vi "Config Axis.vi"(0 "X-Axis configuration":T1, 5 "Y-Axis configuration":T1, 7 "Z-Axis configuration":T1, 11 "error in (no error)":errorcluster) -> (15 "error out":errorcluster)   [LabVIEW 2024, in "GRBL 1.1.lvlib"]
doc: "X-axis travel resolution: X-axis travel resolution in steps per millimeter. (step/mm)\nY-axis travel resolution: Y-axis travel resolution in steps per millimeter. (step/mm)\nZ-axis travel resolution: Z-axis travel resolution in steps per millimeter. (step/mm)\nX-axis maximum rate: X-axis maximum rate. Used as G0 rapid rate. (mm/min)\nY-axis maximum rate: Y-axis maximum rate. Used as G0 rapid rate. (mm/min)\nZ-axis maximum rate: Z-axis maximum rate. Used as G0 rapid rate. (mm/min)\nX-axis acceleration: X-axis acceleration. Used for motion planning to not exceed motor torque and lose steps. (mm/sec^2)\nY-axis acceleration: Y-axis acceleration. Used for motion planning to not exceed motor torque and lose steps. (mm/sec^2)\nZ-axis acceleration: Z-axis acceleration. Used for motion planning to not exceed motor torque and lose steps. (mm/sec^2)\nX-axis maximum travel: Maximum X-axis travel distance from homing switch. Determines valid machine space for soft-limits and homing search distances. (millimeters)\nY-axis maximum travel: Maximum Y-axis travel distance from homing switch. Determines valid machine space for soft-limits and homing search distances. (millimeters)\nZ-axis maximum travel: Maximum Z-axis travel distance from homing switch. Determines valid machine space for soft-limits and homing search distances. (millimeters)"
uses:
  GRBL 1.1.lvlib
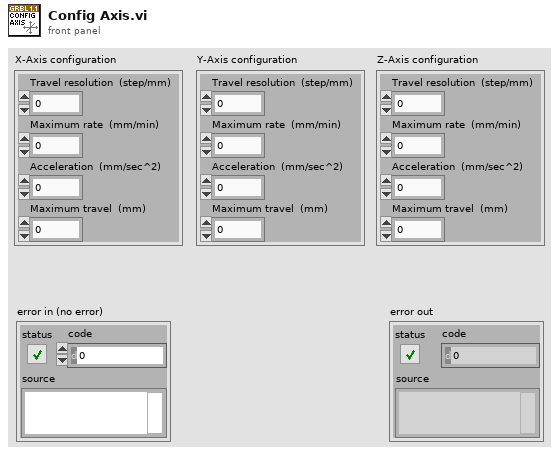
[diagram p1: front panel]
types:
  T1 = cluster{"Travel resolution\t(step/mm)":sgl, "Maximum rate\t(mm/min)":u32, "Acceleration\t(mm/sec^2)":u32, "Maximum travel\t(mm)":u32}
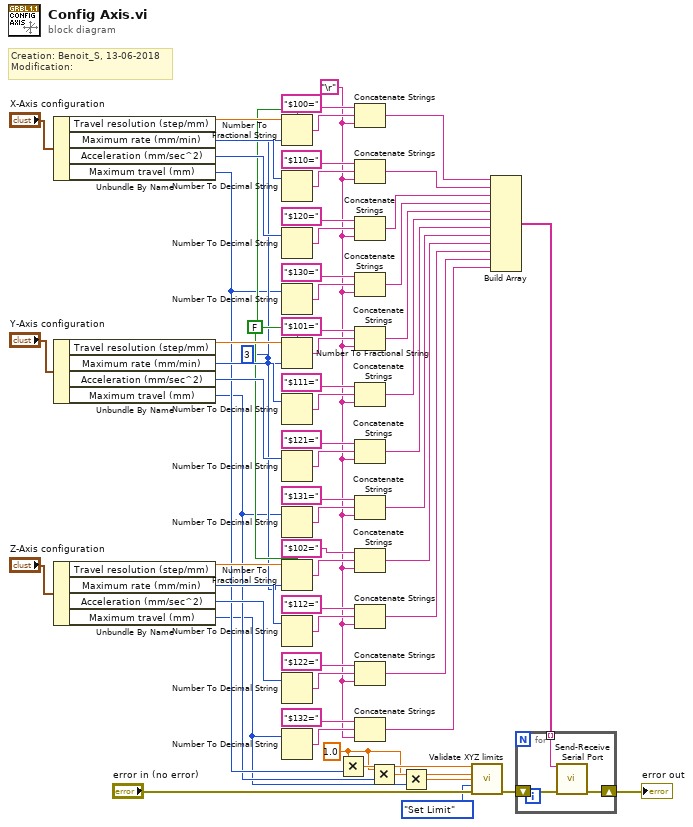
[diagram p0: block diagram]
diagram:
  w2 = sgl 1.0 ("x")
  w26 = FALSE ("use system decimal point (T)")
  w25 = i16 3 ("precision (6)")
  w24 = "\r"
  # "Creation: Benoit_S, 13-06-2018\nModification:"
  n1 = Unbundle By Name("X-Axis configuration") -> ("Travel resolution\t(step/mm)"=w53:sgl, "Maximum rate\t(mm/min)"=w52:u32, "Acceleration\t(mm/sec^2)"=w51:u32, "Maximum travel\t(mm)"=w7:u32)
  n2 = Unbundle By Name("Y-Axis configuration") -> ("Travel resolution\t(step/mm)"=w48:sgl, "Maximum rate\t(mm/min)"=w49:u32, "Acceleration\t(mm/sec^2)"=w50:u32, "Maximum travel\t(mm)"=w6:u32)
  n3 = Unbundle By Name("Z-Axis configuration") -> ("Travel resolution\t(step/mm)"=w32:sgl, "Maximum rate\t(mm/min)"=w31:u32, "Acceleration\t(mm/sec^2)"=w30:u32, "Maximum travel\t(mm)"=w3:u32)
  n4 = Number To Fractional String(use system decimal point (T)=w26, number=w53, precision (6)=w25) -> (F-format string=w60:string)  [unwired: 1 in]
  n5 = Number To Decimal String(number=w52) -> (decimal integer string=w58:string)  [unwired: 1 in]
  n6 = Number To Decimal String(number=w51) -> (decimal integer string=w57:string)  [unwired: 1 in]
  n7 = Number To Decimal String(number=w7) -> (decimal integer string=w54:string)  [unwired: 1 in]
  n8 = Number To Fractional String(use system decimal point (T)=w26, number=w48, precision (6)=w25) -> (F-format string=w41:string)  [unwired: 1 in]
  n9 = Number To Decimal String(number=w49) -> (decimal integer string=w43:string)  [unwired: 1 in]
  n10 = Number To Decimal String(number=w50) -> (decimal integer string=w44:string)  [unwired: 1 in]
  n11 = Number To Decimal String(number=w6) -> (decimal integer string=w47:string)  [unwired: 1 in]
  n12 = Number To Fractional String(use system decimal point (T)=w26, number=w32, precision (6)=w25) -> (F-format string=w39:string)  [unwired: 1 in]
  n13 = Number To Decimal String(number=w31) -> (decimal integer string=w37:string)  [unwired: 1 in]
  n14 = Number To Decimal String(number=w30) -> (decimal integer string=w36:string)  [unwired: 1 in]
  n15 = Number To Decimal String(number=w3) -> (decimal integer string=w33:string)  [unwired: 1 in]
  n16 = Multiply(x=w2, y=w7) -> (x*y=w5:sgl)
  n17 = Concatenate Strings("$100=", w60, w24) -> (w23:string)
  n18 = Concatenate Strings("$110=", w58, w24) -> (w22:string)
  n19 = Concatenate Strings("$120=", w57, w24) -> (w21:string)
  n20 = Concatenate Strings("$130=", w54, w24) -> (w20:string)
  n21 = Concatenate Strings("$101=", w41, w24) -> (w19:string)
  n22 = Concatenate Strings("$111=", w43, w24) -> (w18:string)
  n23 = Concatenate Strings("$121=", w44, w24) -> (w17:string)
  n24 = Concatenate Strings("$131=", w47, w24) -> (w16:string)
  n25 = Concatenate Strings("$102=", w39, w24) -> (w15:string)
  n26 = Concatenate Strings("$112=", w37, w24) -> (w14:string)
  n27 = Concatenate Strings("$122=", w36, w24) -> (w13:string)
  n28 = Concatenate Strings("$132=", w33, w24) -> (w12:string)
  n29 = Multiply(x=w2, y=w6) -> (x*y=w4:sgl)
  n30 = Multiply(x=w2, y=w3) -> (x*y=w1:sgl)
  n31 = call "Validate XYZ limits.vi"("X"=w5, "Y"=w4, "Z"=w1, "Action"=enum16{"Set Limit", "Validate limit"}."Set Limit", "error in (no error)"="error in (no error)") -> ("error out"=w9:errorcluster)  [unwired: 9 in, 1 out]
  n32 = Build Array(w23, w22, w21, w20, w19, w18, w17, w16, w15, w14, w13, w12) -> (w11:string[])
  n33 = for {
    shift-right: [w65] -> w63
    shift-left: w9 -> [w66]
    tunnel: w11 -> [w64] mode=indexing
    n34 = call "Send-Receive Serial Port.vi"("Data to write"=w64, "error in (no error)"=w66) -> ("error out"=w65:errorcluster)  [unwired: 12 in, 1 out]
  }
  "error out" <- w63
